vi "set_increment.vi"(8 "error in (no error)":errorcluster, 9 "time increment":dbl[unit], 10 "z increment":dbl[unit], 11 "DataCollectionDL090215 in":refnum<class "DataCollectionDL090215.lvclass">) -> (0 "error out":errorcluster, 3 "DataCollectionDL090215 out":refnum<class "DataCollectionDL090215.lvclass">)   [LabVIEW 2010, in "DataCollectionDL090215.lvclass"]
uses:
  DataCollectionDL090215.lvclass
  DataCollectionDL090215.lvclass/DataCollectionDL090215.ctl
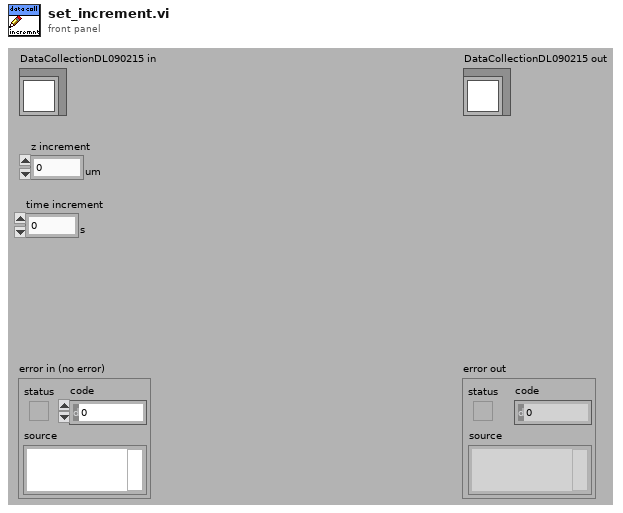
[diagram p1: front panel]
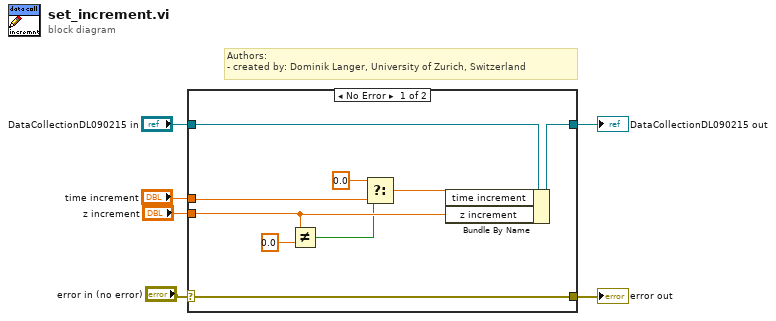
[diagram p0: block diagram]
diagram:
  # "Authors: \n- created by: Dominik Langer, University of Zurich, Switzerland"
  n1 = case shown="No Error" "error in (no error)" {
    selector: "error in (no error)" -> [w15 w16]
    tunnel: [w15 w16] -> w5
    tunnel: [w13 w17] -> w3
    tunnel: "DataCollectionDL090215 in" -> [w14 w17]
    tunnel: "z increment" -> [w12 _]
    tunnel: "time increment" -> [w8 _]
    frame No Error {
      n2 = Not Equal?(x=w12, y=dbl[unit] 0.0) -> (x != y?=w10:bool)
      n3 = Select(t=dbl[unit] 0.0, s=w10, f=w8) -> (s? t:f=w7:dbl[unit])
      n4 = Bundle By Name(cluster=w14, "time increment"=w7, "z increment"=w12) -> (w13:refnum<class "DataCollectionDL090215.lvclass">)
    }
    frame Error {
    }
  }
  "error out" <- w5
  "DataCollectionDL090215 out" <- w3
